vi "To Generic.vi"(8 "error in (no error)":errorcluster, 11 "Enum in":refnum<class "Enum.lvclass">) -> (0 "error out":errorcluster, 2 "Generic Data":refnum<class "Generic Data.lvclass">[](array[class]), 3 "Data Name":string[](array[string]))   [LabVIEW 2020, in "Data.lvlib" / "Enum.lvclass"]
doc: "Present private data as an array of named generic data elements."
uses:
  Enum.lvclass
  Generic Data.lvclass
  Enum.lvclass/Enum.ctl
  U32/U32.lvclass/U32.ctl
  String/String.lvclass/String.ctl
  U32/U32.lvclass
  C:/Users/Henri/OneDrive/LabVIEW/Framework/Data/Generic Data/Generic Data.lvclass
  String/String.lvclass
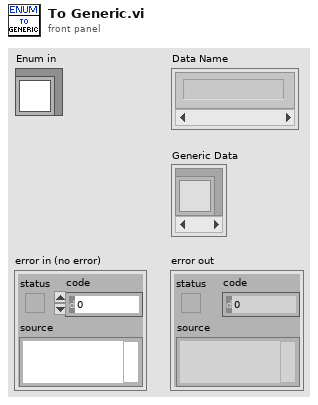
[diagram p1: front panel]
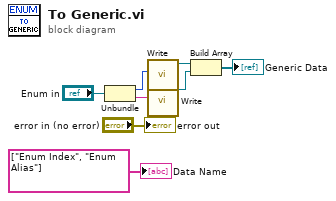
[diagram p0: block diagram]
diagram:
  n1 = Unbundle("Enum in") -> (w7:u32, w6:string)
  n2 = call "Write.vi"("U32"=w7) -> ("U32 out"=w5:refnum<class "U32.lvclass">)  [unwired: 10 in]
  n3 = call "Write.vi"("String"=w6) -> ("String out"=w4:refnum<class "String.lvclass">)  [unwired: 10 in]
  n4 = Build Array(w5, w4) -> (→"Generic Data":refnum<class "Generic Data.lvclass">[])
  "error out" <- "error in (no error)"
  "Data Name" <- string[] ["Enum Index", "Enum Alias"] ("Data Name")
